vi "Data.Engine.Initialize.vi"(8 "error in":errorcluster, 11 "Custom Device Ref":T1 format="%.0x") -> (0 "error out":errorcluster, 2 "Data Access Engine":refnum<class "Data Access Engine.lvclass">, 3 "Custom Device Ref":T1 format="%.0x")   [LabVIEW 2015, in "Data Access Engine.lvlib" / "Data Access Engine.lvclass"]
uses:
  Data Access Engine.lvclass
  <vilib>/NI Veristand/Custom Device API/Custom Device Item Ref.ctl
  <vilib>/NI Veristand/Custom Device API/Block Data Reference.ctl
  <vilib>/NI Veristand/Custom Device API/Data Reference.ctl
  Access Type Classes/Read/Read.lvclass
  Access Type Classes/Write/Write.lvclass
  Access Type Classes/ReadWrite/ReadWrite.lvclass
  Data Access Engine.lvclass/Data Access Engine.ctl
  <vilib>/NI Veristand/Custom Device API/Get Item Property (Variant).vi
  <vilib>/NI Veristand/Custom Device API/Custom Device API.lvlib
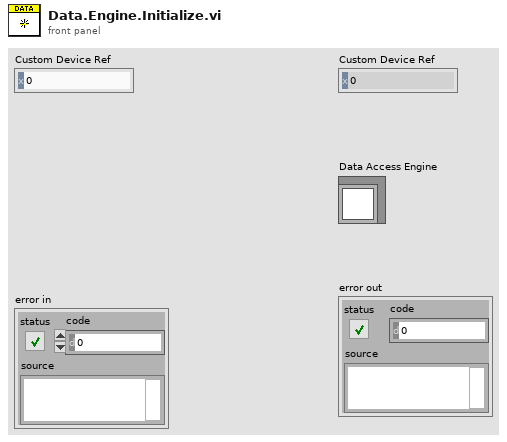
[diagram p1: front panel]
types:
  T1 = typedef "Custom Device API.lvlib/Custom Device Item Ref.ctl" = u64
  T2 = typedef "Custom Device API.lvlib/Block Data Reference.ctl" = cluster{"Data Reference":T3, "Offset":u64, "Length":u64}
  T3 = typedef "Custom Device API.lvlib/Data Reference.ctl" = i32
  T4 = cluster{"Read":cluster{"Refs":T2[], "Values":dbl[]}[], "Write":cluster{"Refs":T3[], "Values":dbl[]}[], "ReadWrite":cluster{"Refs":T3[], "Values":dbl[], "Reset Values":dbl[]}[], "LUT":variant}
  T5 = cluster{"Refs":T3[], "Values":dbl[], "Reset Values":dbl[]}[]
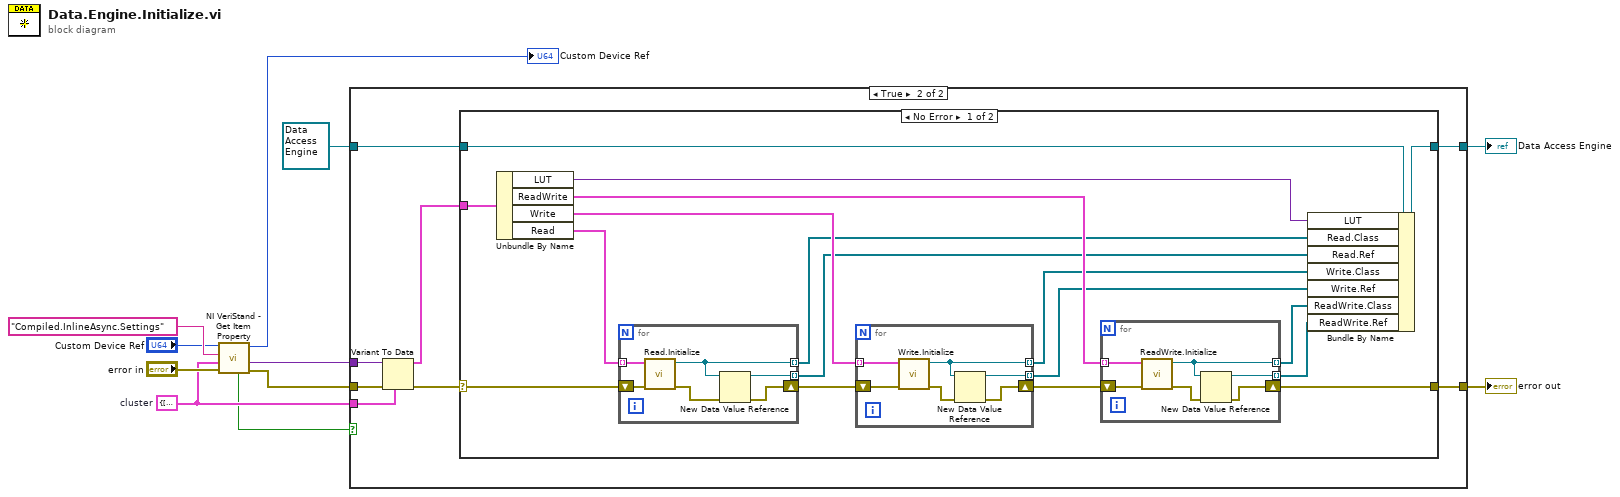
[diagram p0: block diagram]
diagram:
  w7 = T4 {"Read"=[], "Write"=[], "ReadWrite"=[], "LUT"=variant}  # cluster
  n1 = call-poly <vilib>:"NI VeriStand - Get Item Property.vi"("error in (no error)"="error in", "Default Value"=w7, "Property Name"="Compiled.InlineAsync.Settings", "Item Ref in"="Custom Device Ref") -> ("error out"=w10:errorcluster, "Value"=w8:variant, "Item Ref out"=→"Custom Device Ref":T1, "Found?"=w1:bool)  [unwired: 4 in]
  n2 = case shown="True" w1 {
    tunnel: w10 -> [w12 w21]
    tunnel: w8 -> [_ w20]
    tunnel: w7 -> [_ w19]
    tunnel: [w13 w18] -> w6
    tunnel: refnum<class "Data Access Engine.lvclass"> refnum ("Data Access API.lvlib:Data Access API.lvclass") -> [w13 w16]
    tunnel: [w12 w14] -> w4
    frame False {
    }
    frame True {
      n3 = Variant To Data(error in=w21, type=w19, Variant=w20) -> (data=w17:T4, error out=w15:errorcluster)
      n4 = case shown="No Error" w15 {
        selector: w15 -> [w37 w58]
        tunnel: [w34 w58] -> w14
        tunnel: [w28 w57] -> w18
        tunnel: w16 -> [w23 w57]
        tunnel: w17 -> [w24 _]
        frame No Error {
          n5 = Unbundle By Name(w24) -> ("LUT"=w22:variant, "ReadWrite"=w32:T5, "Write"=w33:cluster{"Refs":T3[], "Values":dbl[]}[], "Read"=w38:cluster{"Refs":T2[], "Values":dbl[]}[])
          n6 = for {
            tunnel: w38 -> [w56] mode=indexing
            shift-right: [w53] -> w36
            shift-left: w37 -> [w55]
            tunnel: [w52] -> w29 mode=indexing
            tunnel: [w51] -> w25 mode=indexing
            n7 = call "Read.Initialize.vi"("error in (no error)"=w55, "Settings"=w56) -> ("error out"=w54:errorcluster, "Read out"=w52:refnum<class "Read.lvclass">)  [unwired: 8 in]
            n8 = New Data Value Reference(data value=w52, error in=w54) -> (data value reference=w51:refnum<data-value>, error out=w53:errorcluster)
          }
          n9 = for {
            tunnel: w33 -> [w50] mode=indexing
            shift-right: [w46] -> w35
            shift-left: w36 -> [w49]
            tunnel: [w48] -> w30 mode=indexing
            tunnel: [w45] -> w26 mode=indexing
            n10 = call "Write.Initialize.vi"("error in (no error)"=w49, "Settings"=w50) -> ("error out"=w47:errorcluster, "Write out"=w48:refnum<class "Write.lvclass">)  [unwired: 8 in]
            n11 = New Data Value Reference(data value=w48, error in=w47) -> (data value reference=w45:refnum<data-value>, error out=w46:errorcluster)
          }
          n12 = for {
            tunnel: w32 -> [w43] mode=indexing
            shift-right: [w41] -> w34
            shift-left: w35 -> [w44]
            tunnel: [w40] -> w31 mode=indexing
            tunnel: [w39] -> w27 mode=indexing
            n13 = call "ReadWrite.Initialize.vi"("error in (no error)"=w44, "Settings"=w43) -> ("error out"=w42:errorcluster, "ReadWrite out"=w40:refnum<class "ReadWrite.lvclass">)  [unwired: 8 in]
            n14 = New Data Value Reference(data value=w40, error in=w42) -> (data value reference=w39:refnum<data-value>, error out=w41:errorcluster)
          }
          n15 = Bundle By Name(cluster=w23, "LUT"=w22, "Read.Class"=w29, "Read.Ref"=w25, "Write.Class"=w30, "Write.Ref"=w26, "ReadWrite.Class"=w31, "ReadWrite.Ref"=w27) -> (w28:refnum<class "Data Access Engine.lvclass">)
        }
        frame Error {
        }
      }
    }
  }
  "error out" <- w4
  "Data Access Engine" <- w6
